vi "Save All Error Codes Files.vi"(7 "scope":T1, 8 "error in (no error)":errorcluster, 10 "save? (T)":bool=TRUE, 11 "error list <top>":variant) -> (0 "error out":errorcluster)   [LabVIEW 2017]
uses:
  Error List/Scope.ctl
  Error File Management/Error File Management.lvlib
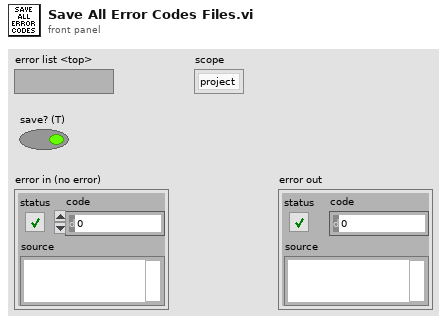
[diagram p1: front panel]
types:
  T1 = typedef "Scope.ctl" = enum16{"project", "global"}
  T2 = typedef "Error Code File Properties.ctl" = cluster{"path":path, "simplified path":string, "name":string, "display name":string, "family name":string, "comment":string, "parsable?":bool, "file modified?":bool}
  T3 = typedef "Error File Management.lvlib/NI Error.ctl" = errorcluster
  T4 = cluster{"family name":string, "display name":string}
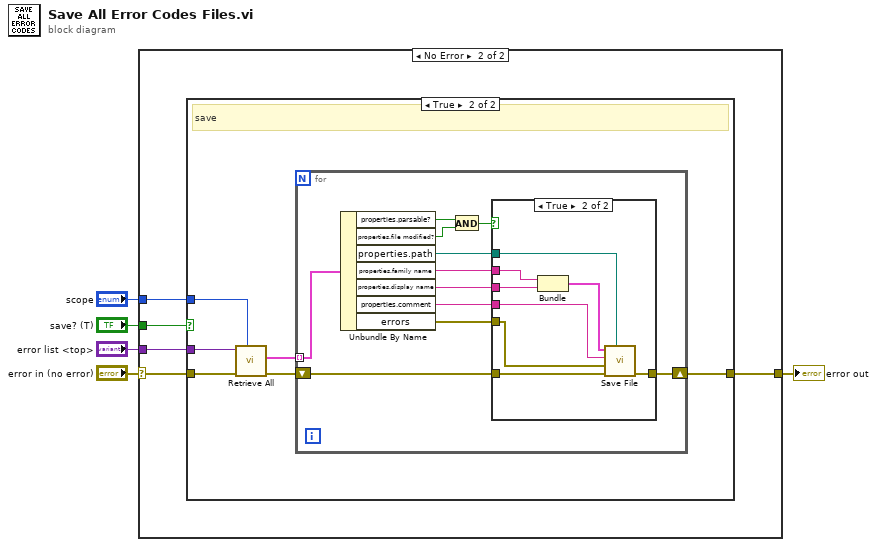
[diagram p0: block diagram]
diagram:
  n1 = case shown="No Error" "error in (no error)" {
    selector: "error in (no error)" -> [w6 w10]
    tunnel: "save? (T)" -> [_ w11]
    tunnel: [w6 w9] -> w3
    tunnel: "error list <top>" -> [_ w8]
    tunnel: "scope" -> [_ w7]
    frame Error {
    }
    frame No Error {
      n2 = case shown="True" w11 {
        tunnel: w10 -> [w12 w18]
        tunnel: [w12 w17] -> w9
        tunnel: w8 -> [_ w16]
        tunnel: w7 -> [_ w15]
        frame False {
          # "not save"
        }
        frame True {
          # "save"
          n3 = call "Retrieve All.vi"("scope"=w15, "error in (no error)"=w18, "error list <top>"=w16) -> ("error out"=w14:errorcluster, "error list content"=w13:cluster{"properties":T2, "errors":T3[]}[])  [unwired: 6 in, 1 out]
          n4 = for {
            shift-right: [w24] -> w17
            shift-left: w14 -> [w25]
            tunnel: w13 -> [w23] mode=indexing
            n5 = Unbundle By Name(w23) -> ("properties.parsable?"=w20:bool, "properties.file modified?"=w21:bool, "properties.path"=w29:path, "properties.family name"=w28:string, "properties.display name"=w27:string, "properties.comment"=w26:string, "errors"=w22:T3[])
            n6 = And(x=w20, y=w21) -> (x .and. y?=w19:bool)
            n7 = case shown="True" w19 {
              tunnel: w29 -> [_ w33]
              tunnel: w28 -> [_ w36]
              tunnel: w27 -> [_ w35]
              tunnel: w26 -> [_ w32]
              tunnel: w25 -> [w30 w38]
              tunnel: [w30 w37] -> w24
              tunnel: w22 -> [_ w31]
              frame False {
              }
              frame True {
                n8 = Bundle("family name"=w36, "display name"=w35) -> (w34:T4)  [unwired: 1 in]
                n9 = call "Save File.vi"("error codes file"=w33, "error in (no error)"=w38, "errors"=w31, "comment"=w32, "family"=w34) -> ("error out"=w37:errorcluster)  [unwired: 6 in]
              }
            }
          }
        }
      }
    }
  }
  "error out" <- w3
